vi "Read Base Description.vi"(11 "Condiment Decorator in":refnum<class "Condiment Decorator.lvclass">) -> (2 "String":string)   [LabVIEW 2013, in "Condiment Decorator.lvclass"]
uses:
  Condiment Decorator.lvclass
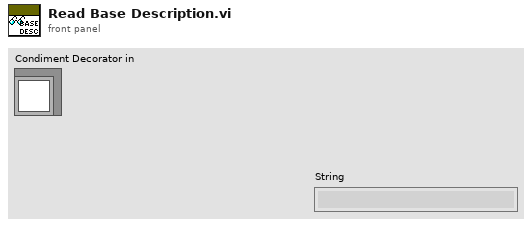
[diagram p1: front panel]
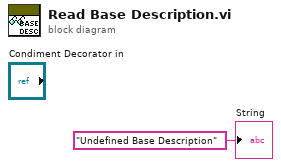
[diagram p0: block diagram]
diagram:
  "String" <- "Undefined Base Description" ("String")
